vi "CAN Initialize.vi"(8 "错误输入（无错误）":errorcluster, 10 "Btr0Btr1":u16=28 format="%.0x", 11 "Channel":u16=81 format="%.0x") -> (0 "错误输出":errorcluster, 2 "Channel out":u16, 3 "function return":u32 format="%.0x")   [LabVIEW 2021, in "PCANBasic.lvlib"]
doc: "TPCANStatus __stdcall CAN_Initialize(\n TPCANHandle Channel, \n TPCANBaudrate Btr0Btr1, \n TPCANType HwType _DEF_ARG,\n DWORD IOPort _DEF_ARG, \n WORD Interrupt _DEF_ARG);"
uses:
  <userlib>/PCANBasic/PCANBasic.lvlib
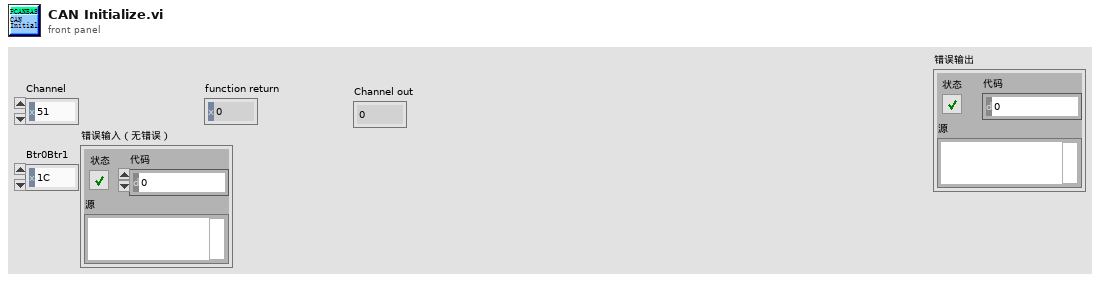
[diagram p1: front panel]
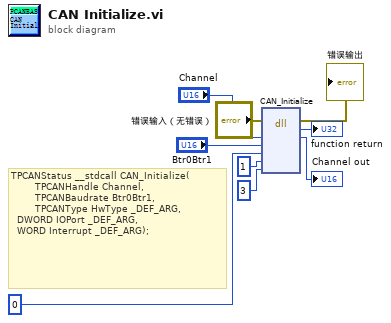
[diagram p0: block diagram]
diagram:
  # "TPCANStatus __stdcall CAN_Initialize(\n        TPCANHandle Channel, \n        TPCANBaudrate Btr0Btr1, \n        TPCANType HwType _DEF_ARG,\n\t\tDWORD IOPort _DEF_ARG, \n\t\tWORD Interrupt _DEF_ARG);"
  n1 = dll-call lib="PTH2gabs CUsersAdministrator.CH-202202160008Desktop电流传感器测试\tdll文件\nPCANBasic.dll" fn="CAN_Initialize"(error in="错误输入（无错误）", "Channel"="Channel", "Btr0Btr1"="Btr0Btr1", "TPCANtype"=u8 0, "IOport"=u32 1, "interrupt"=u16 3) -> (error out=→"错误输出":errorcluster, "返回类型"=→"function return":u32, "Channel"=→"Channel out":u16)  [unwired: 6 in, 1 out]
